vi "Import Configuration RTM.vi"(8 "error in (no error)":errorcluster, 11 "Node Ptr":u64 format="%.0x") -> (0 "error out":errorcluster)   [LabVIEW 2020, in "Routing and Faulting System Explorer.lvlib"]
uses:
  Routing and Faulting System Explorer.lvlib
  Scripting/Routing and Faulting Scripting.lvlib
panel:
  in  "Path":path
  in  "Tag":string
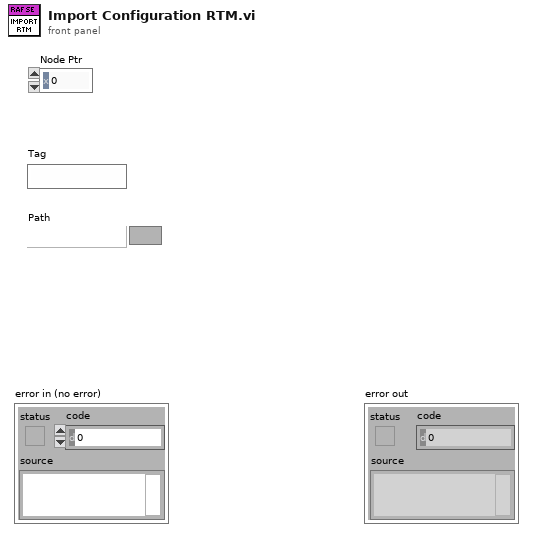
[diagram p1: front panel]
types:
  T1 = typedef "Custom Device API.lvlib/Custom Device Item Ref.ctl" = u64
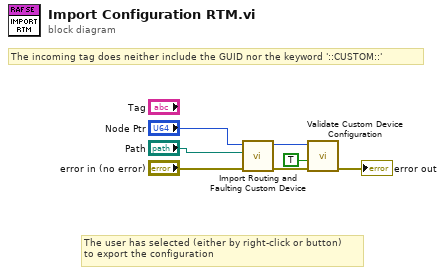
[diagram p0: block diagram]
diagram:
  # "The user has selected (either by right-click or button)\nto export the configuration"
  # "The incoming tag does neither include the GUID nor the keyword '::CUSTOM::'"
  n1 = call "Import Routing and Faulting Custom Device.vi"("error in"="error in (no error)", "datalog path (use dialog)"="Path", "routing and faulting custom device in"="Node Ptr") -> ("error out"=w5:errorcluster, "routing and faulting custom device out"=w2:T1)  [unwired: 7 in]
  n2 = call "Validate Custom Device Configuration.vi"("error in (no error)"=w5, "Force Validation (F)"=TRUE, "Routing and Faulting Custom Device Ref"=w2) -> ("error out"=→"error out":errorcluster)  [unwired: 6 in, 2 out]
